vi "Setup.vi"(9 "Active Project":refnum<vi>, 10 "NI.LV.Dialog Instance":refnum<vi>) -> (2 "Found Target":string, 3 "_Rescript Msg out":refnum<class "_Msg Rescript.lvclass">)   [LabVIEW 2025, in "_Msg Rescript.lvlib" / "_Msg Rescript.lvclass"]
uses:
  _Msg Rescript.lvclass
  _Msg Rescript.lvclass/_Msg Rescript.ctl
  _Shared/Project Stuff/Project Stuff.lvclass
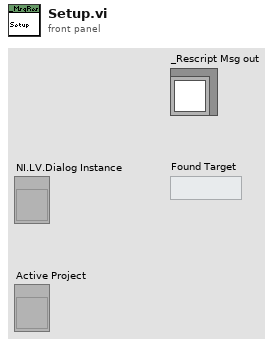
[diagram p1: front panel]
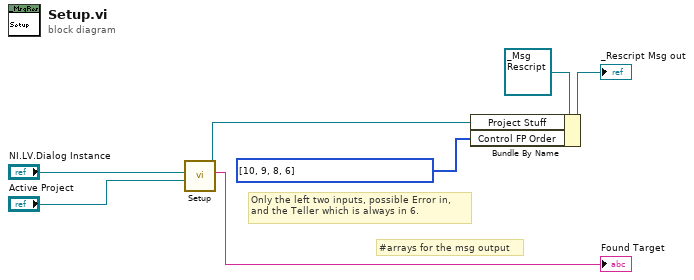
[diagram p0: block diagram]
diagram:
  # "#arrays for the msg output"
  # "Only the left two inputs, possible Error in, and the Teller which is always in 6."
  n1 = call "Setup.vi"("Active Project"="Active Project", "NI.LV.Dialog Instance"="NI.LV.Dialog Instance") -> ("Found Target"=→"Found Target":string, "Project Stuff out"=w2:refnum<class "Project Stuff.lvclass">)  [unwired: 8 in]
  n2 = Bundle By Name(cluster=refnum<class "_Msg Rescript.lvclass"> refnum ("_Rescript Msg out"), "Project Stuff"=w2, "Control FP Order"=i32[] [10, 9, 8, 6]) -> (→"_Rescript Msg out":refnum<class "_Msg Rescript.lvclass">)
